vi "FormLogin.vi"() -> ()   [LabVIEW 2013]
uses:
  <vilib>/addons/database/_DB Variant To Data/Database Variant To Data.xnode
panel:
  out "管理员":string(combo)
  out "编号":string(combo)
  in  "联机模式":enum32{"未选择", "联网模式", "单机模式"}(radio)
  in  "用户登录":bool
  out "udl名称":string="epsacc.udl"
  in  "修改密码":bool
  in  "用户名":string(combo)
  in  "密码":string
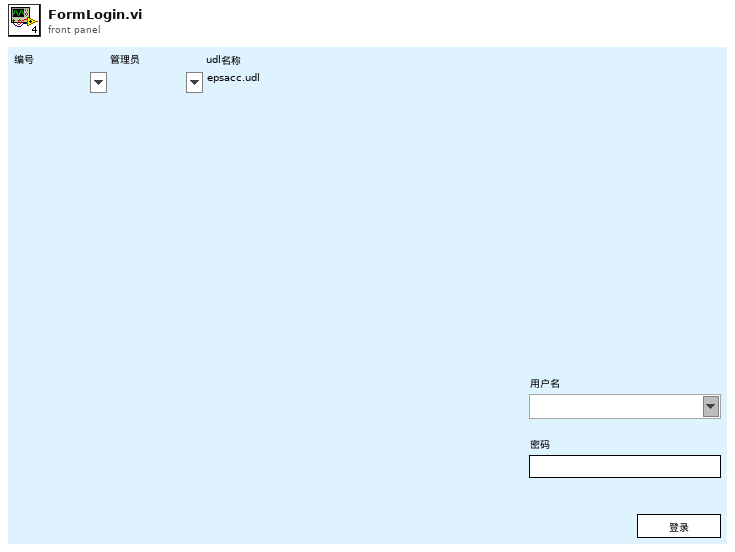
[diagram p1: front panel]
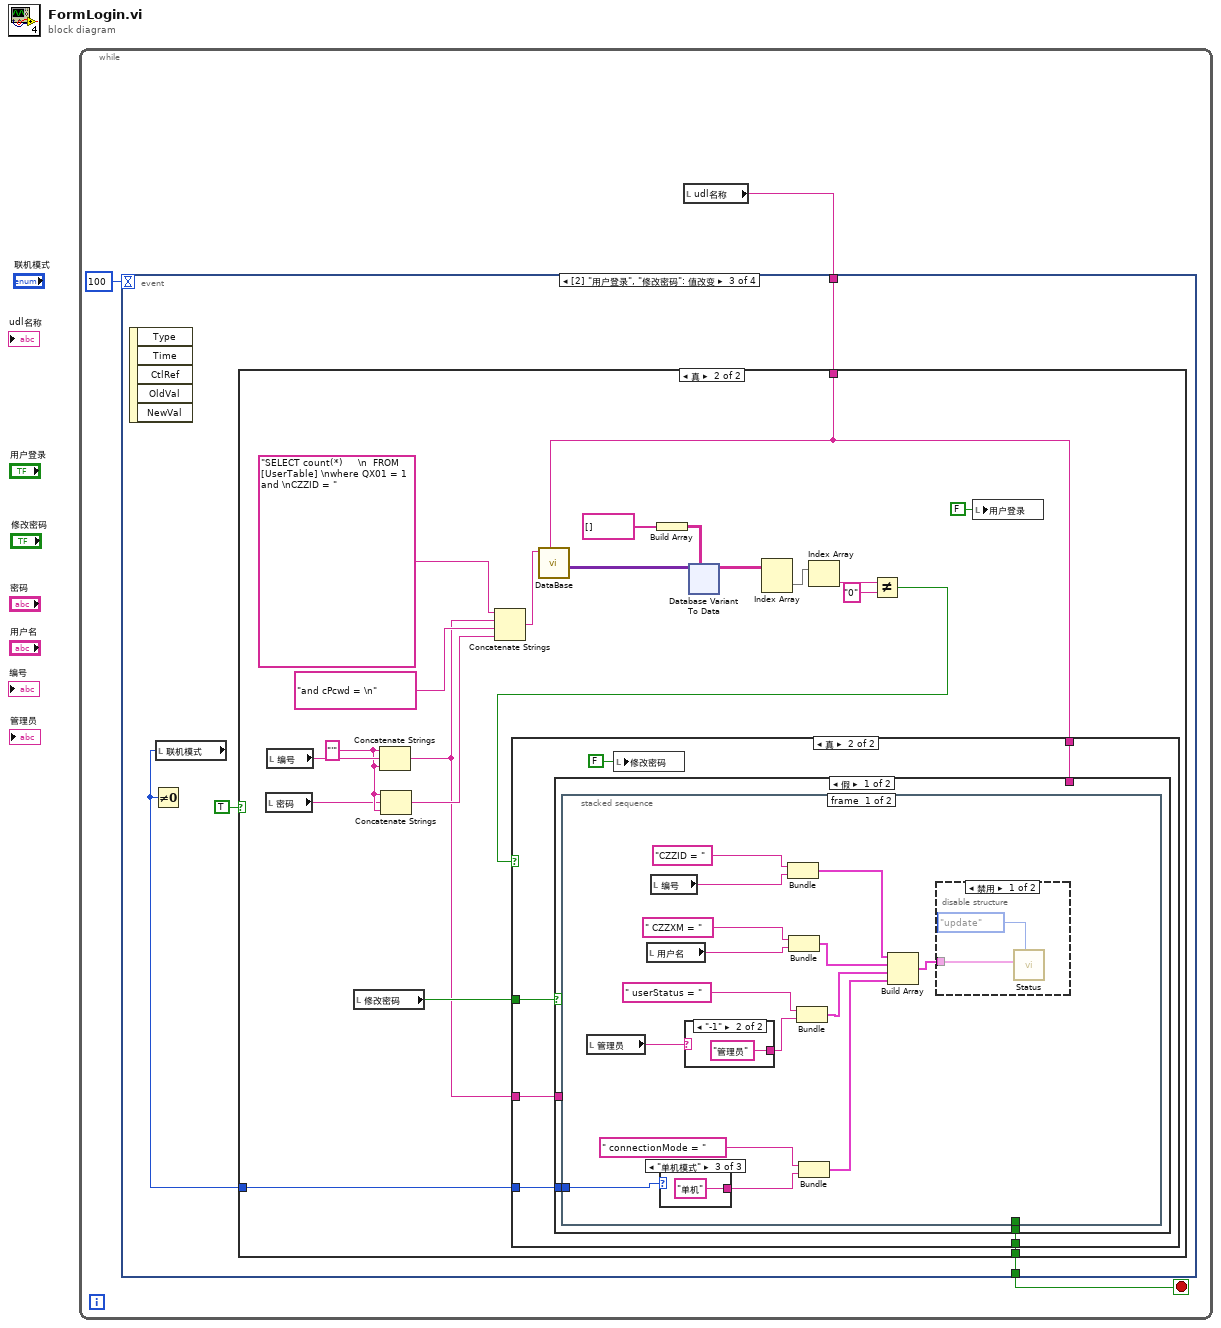
[diagram p0: block diagram]
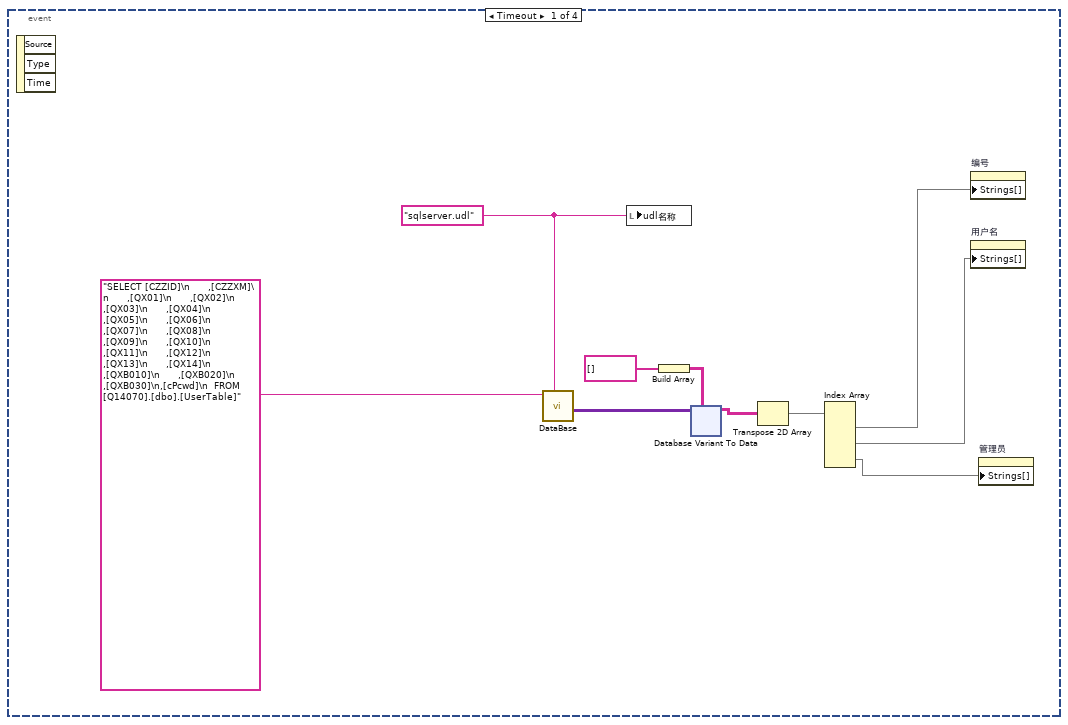
[diagram p2: hidden frame]
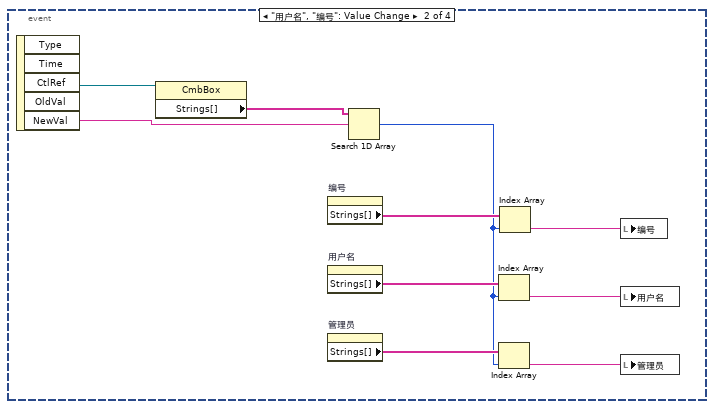
[diagram p3: hidden frame]
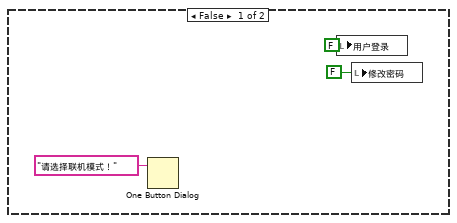
[diagram p4: hidden frame]
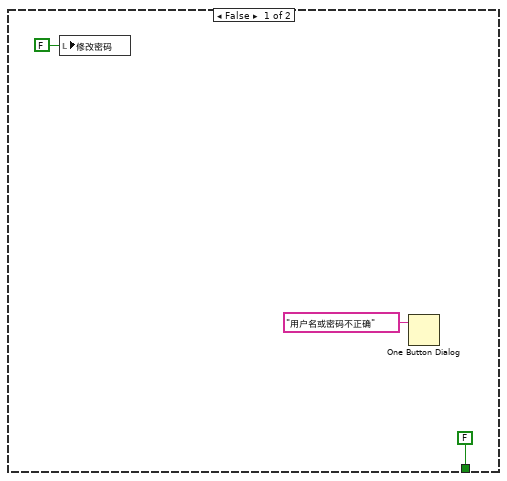
[diagram p5: hidden frame]
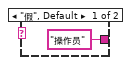
[diagram p7: hidden frame]
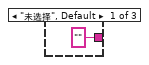
[diagram p8: hidden frame]
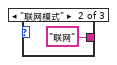
[diagram p9: hidden frame]
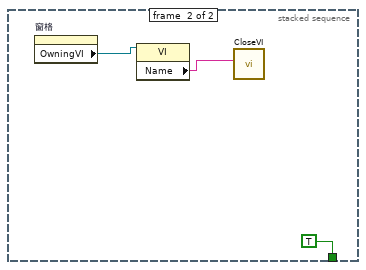
[diagram p10: hidden frame]
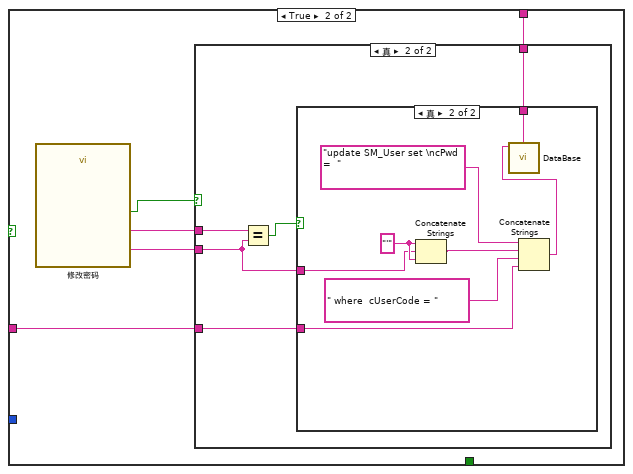
[diagram p11: hidden frame]
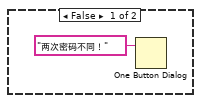
[diagram p13: hidden frame]
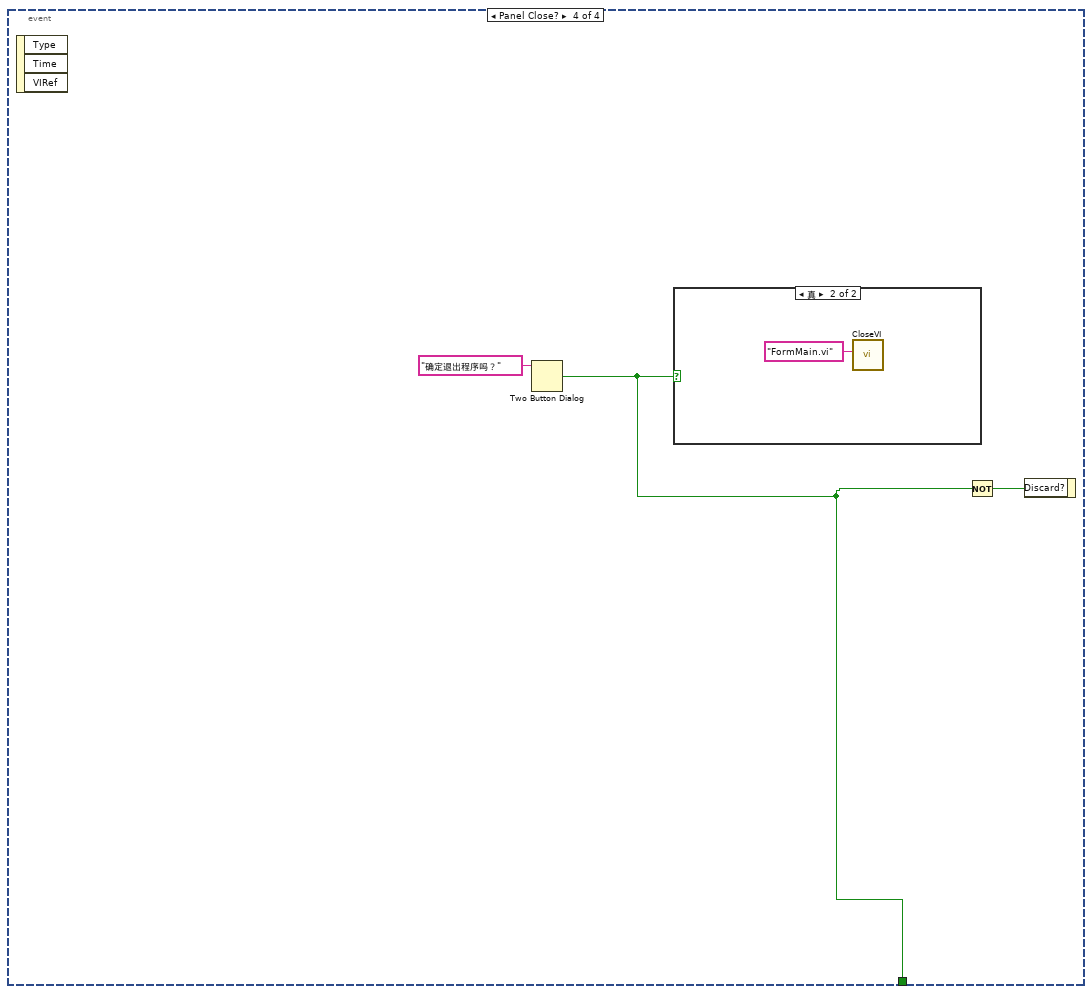
[diagram p14: hidden frame]
diagram:
  n1 = while {
    stop <- w3 stop-if-true
    n2 = local read "udl名称"() -> (w1:string)
    n3 = event shown="[2] \"用户登录\", \"修改密码\": 值改变" {
      selector: _ -> [_ _ _ _]
      dyn-events: _ -> [_ _ _ _]
      timeout: 100 -> [_ _ _ _]
      tunnel: [_ _ w71 w195] -> w3
      tunnel: w1 -> [_ _ w69 _]
      event Timeout {
        w4 = "sqlserver.udl" ("udl名称")
        n4 = event-data() -> ()  [unwired: 1 in, 3 out]
        n5 = call "DataBase.vi"("udl名称"=w4, "SQL query"="SELECT [CZZID]\n      ,[CZZXM]\n      ,[QX01]\n      ,[QX02]\n      ,[QX03]\n      ,[QX04]\n      ,[QX05]\n      ,[QX06]\n      ,[QX07]\n      ,[QX08]\n      ,[QX09]\n      ,[QX10]\n      ,[QX11]\n      ,[QX12]\n      ,[QX13]\n      ,[QX14]\n      ,[QXB010]\n      ,[QXB020]\n      ,[QXB030]\n,[cPcwd]\n  FROM [Q14070].[dbo].[UserTable]") -> ("recordset data"=w6:variant[][])  [unwired: 9 in]
        n6 = local write "udl名称"(w4) -> ()
        n7 = Build Array(string[] [] ("添加的数组")) -> (w8:string[][])
        n8 = xnode "Database Variant To Data"("database variant"=w6, "type"=w8) -> ("data"=w7:string[][])  [unwired: 1 in, 1 out]
        n9 = Transpose 2D Array(2D array=w7) -> (transposed array=w5:string[][])
        n10 = Index Array(array=w5) -> (element #1=w13:string[], element #2=w11:string[], element #3=w10:string[])  [unwired: 6 in]
        n11 = property on="编号" class="CmbBox"("Strings[]"=w13) -> ()  [unwired: 2 in, 2 out]
        n12 = property on="用户名" class="CmbBox"("Strings[]"=w11) -> ()  [unwired: 2 in, 2 out]
        n13 = property on="管理员" class="CmbBox"("Strings[]"=w10) -> ()  [unwired: 2 in, 2 out]
      }
      event "用户名", "编号": Value Change {
        n14 = event-data() -> ("CtlRef"=w67:refnum<vi>, "NewVal"=w65:string)  [unwired: 1 in, 3 out]
        n15 = property class="CmbBox"(reference=w67) -> ("Strings[]"=w66:string[])  [unwired: 1 in, 2 out]
        n16 = property on="编号" class="CmbBox"() -> ("Strings[]"=w64:string[])  [unwired: 2 in, 2 out]
        n17 = property on="用户名" class="CmbBox"() -> ("Strings[]"=w63:string[])  [unwired: 2 in, 2 out]
        n18 = property on="管理员" class="CmbBox"() -> ("Strings[]"=w59:string[])  [unwired: 2 in, 2 out]
        n19 = Search 1D Array(1D array=w66, element=w65) -> (index of element=w58:i32)  [unwired: 1 in]
        n20 = Index Array(array=w63, index=w58) -> (element=w61:string)
        n21 = Index Array(array=w59, index=w58) -> (element=w60:string)
        n22 = Index Array(array=w64, index=w58) -> (element=w62:string)
        n23 = local write "编号"(w62) -> ()
        n24 = local write "用户名"(w61) -> ()
        n25 = local write "管理员"(w60) -> ()
      }
      event "用户登录", "修改密码": Value Change {
        n26 = event-data() -> ()  [unwired: 1 in, 5 out]
        n27 = local read "联机模式"() -> (w70:enum32{"未选择", "联网模式", "单机模式"})
        n28 = Not Equal To 0?(x=w70) -> ()  [unwired: 1 out]
        n29 = case shown="真" TRUE {
          tunnel: [_ w95] -> w71
          tunnel: w69 -> [_ w75]
          tunnel: w70 -> [_ w77]
          frame False {
            n30 = One Button Dialog(message="请选择联机模式！" ("消息")) -> ()  [unwired: 1 in, 1 out]
            n31 = local write "用户登录"(FALSE ("登录")) -> ()
            n32 = local write "修改密码"(FALSE ("登录")) -> ()
          }
          frame True {
            w90 = "'"
            n33 = local read "密码"() -> (w89:string)
            n34 = local read "编号"() -> (w91:string)
            n35 = local read "修改密码"() -> (w83:bool)
            n36 = Concatenate Strings(w90, w91, w90) -> (w76:string)
            n37 = Concatenate Strings(w90, w89, w90) -> (w86:string)
            n38 = Concatenate Strings("SELECT count(*)     \n  FROM [UserTable] \nwhere QX01 = 1 and \nCZZID = " ("SQL query"), w76, "and cPcwd = \n" ("SQL query"), w86) -> (w85:string)
            n39 = call "DataBase.vi"("udl名称"=w75, "SQL query"=w85) -> ("recordset data"=w92:variant[][])  [unwired: 9 in]
            n40 = Build Array(string[] [] ("添加的数组")) -> (w93:string[][])
            n41 = xnode "Database Variant To Data"("database variant"=w92, "type"=w93) -> ("data"=w84:string[][])  [unwired: 1 in, 1 out]
            n42 = Index Array(array=w84) -> (element=w82:string[])  [unwired: 2 in]
            n43 = Index Array(array=w82) -> (element=w81:string)  [unwired: 1 in]
            n44 = Not Equal?(x=w81, y="0") -> (x != y?=w79:bool)
            n45 = case shown="真" w79 {
              tunnel: [FALSE w148] -> w95
              tunnel: w83 -> [_ w147]
              tunnel: w77 -> [_ w145]
              tunnel: w76 -> [_ w144]
              tunnel: w75 -> [_ w143]
              frame False {
                n46 = local write "修改密码"(FALSE ("登录")) -> ()
                n47 = One Button Dialog(message="用户名或密码不正确" ("消息")) -> ()  [unwired: 1 in, 1 out]
              }
              frame True {
                n48 = case shown="假" w147 {
                  tunnel: [w150 _] -> w148
                  tunnel: w145 -> [w149 _]
                  tunnel: w144 -> [_ w177]
                  tunnel: w143 -> [_ w176]
                  frame False {
                    n49 = stacked-sequence {
                      tunnel: [_ TRUE] -> w150
                      tunnel: w149 -> [w165 _]
                      frame #0 {
                        n50 = local read "管理员"() -> (w164:string)
                        n51 = local read "用户名"() -> (w160:string)
                        n52 = local read "编号"() -> (w162:string)
                        n53 = case shown="\"单机模式\"" w165 {
                          tunnel: ["" "联网" "单机"] -> w157
                          frame "未选择", Default {
                          }
                          frame "联网模式" {
                          }
                          frame "单机模式" {
                          }
                        }
                        n54 = case shown="\"-1\"" w164 {
                          tunnel: ["操作员" "管理员"] -> w159
                          frame "假", Default {
                          }
                          frame "-1" {
                          }
                        }
                        n55 = Bundle("y"="CZZID = ", "编号"=w162) -> (w155:cluster{"y":string, "编号":string})  [unwired: 1 in]
                        n56 = Bundle("y"=" CZZXM = ", "用户名"=w160) -> (w154:cluster{"y":string, "用户名":string})  [unwired: 1 in]
                        n57 = Bundle("y"=" userStatus = ", w159) -> (w153:cluster{"y":string, string})  [unwired: 1 in]
                        n58 = Bundle("y"=" connectionMode = ", w157) -> (w152:cluster{"y":string, string})  [unwired: 1 in]
                        n59 = Build Array(w155, w154, w153, w152) -> (w151:cluster{"y":string, "用户名":string}[])
                        n60 = disable-structure shown="禁用" {
                          disable-tunnel: w151 -> [w166 _]
                          frame Disabled {
                            n61 = call "Status.vi"("模式"=enum16{"select", "insert", "update", "delete"}."update", "nameData"=w166) -> ()  [unwired: 9 in, 1 out]
                          }
                          frame Enabled {
                          }
                        }
                      }
                      frame #1 {
                        n62 = property on="窗格" class="Pane"() -> ("OwningVI"=w174:refnum<vi>)  [unwired: 2 in, 2 out]
                        n63 = property class="VI"(reference=w174) -> ("Name"=w173:string)  [unwired: 1 in, 2 out]
                        n64 = call "CloseVI.vi"("名称或相对路径"=w173) -> ()  [unwired: 10 in, 1 out]
                      }
                    }
                  }
                  frame True {
                    n65 = call "修改密码"() -> ("确认密码"=w178:string, "新密码"=w179:string, "确定"=w180:bool)  [unwired: 16 in, 1 out]
                    n66 = case shown="真" w180 {
                      tunnel: w179 -> [_ w185]
                      tunnel: w178 -> [_ w182]
                      tunnel: w176 -> [_ w183]
                      tunnel: w177 -> [_ w181]
                      frame False {
                      }
                      frame True {
                        n67 = Equal?(x=w185, y=w182) -> (x = y?=w184:bool)
                        n68 = case shown="真" w184 {
                          tunnel: w183 -> [_ w194]
                          tunnel: w182 -> [_ w187]
                          tunnel: w181 -> [_ w191]
                          frame False {
                            n69 = One Button Dialog(message="两次密码不同！" ("消息")) -> ()  [unwired: 1 in, 1 out]
                          }
                          frame True {
                            w189 = "'"
                            n70 = Concatenate Strings(w189, w187, w189) -> (w188:string)
                            n71 = Concatenate Strings("update SM_User set \ncPwd =  " ("SQL query"), w188, " where  cUserCode = " ("SQL query"), w191) -> (w190:string)
                            n72 = call "DataBase.vi"("udl名称"=w194, "SQL query"=w190) -> ()  [unwired: 9 in, 1 out]
                          }
                        }
                      }
                    }
                  }
                }
                n73 = local write "修改密码"(FALSE ("登录")) -> ()
              }
            }
            n74 = local write "用户登录"(FALSE ("登录")) -> ()
          }
        }
      }
      event Panel Close? {
        n75 = event-data() -> ()  [unwired: 1 in, 3 out]
        n76 = Two Button Dialog(message="确定退出程序吗？" ("消息")) -> (T button?=w195:bool)  [unwired: 2 in]
        n77 = case shown="真" w195 {
          frame False {
          }
          frame True {
            n78 = call "CloseVI.vi"("名称或相对路径"="FormMain.vi") -> ()  [unwired: 10 in, 1 out]
          }
        }
        n79 = Not(x=w195) -> (.not. x?=w196:bool)
        n80 = event-data("Discard?"=w196) -> ()  [unwired: 1 in, 1 out]
      }
    }
  }
